vi "Configurator.vi"() -> ()   [LabVIEW 2017]
uses:
  Controls/Configurator Range Enum Type Def.ctl
  Controls/Configurator Rate Enum Type Def.ctl
  Controls/Configurator Resolution Enum Type Def.ctl
  Controls/Configurator State Type Def.ctl
panel:
  in  "Baud":bool=TRUE
  in  "First Erase?":bool=TRUE
  in  "VISA Port":refnum<visa-resource-name>="COM5"
  out "Error Out":errorcluster
  in  "Error In":errorcluster
  in  "Resolution":T1=enum."High Res (12 bit)"
  in  "ID":u8
  in  "Rate":T2
  in  "Range":T3=enum."±2g"
  # "Read and save measurement data before running this program!"
  # "6 Meg"
  # "3 Meg"
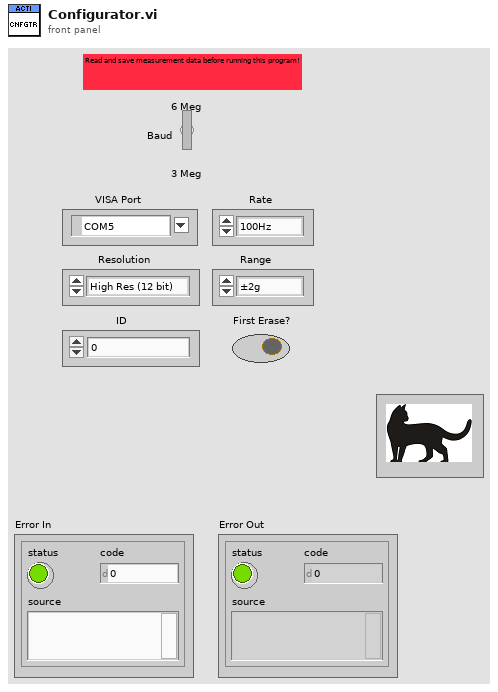
[diagram p1: front panel]
types:
  T1 = typedef "Configurator Resolution Enum Type Def.ctl" = enum16{"Low Res (10 bit)", "High Res (12 bit)"}
  T2 = typedef "Configurator Rate Enum Type Def.ctl" = enum16{"100Hz", "50Hz", "25Hz", "10Hz", "1Hz", "Idle"}
  T3 = typedef "Configurator Range Enum Type Def.ctl" = enum16{"±16g", "±8g", "±4g", "±2g"}
  T4 = typedef "Configurator State Type Def.ctl" = enum16{"Send Idle", "Send Time", "Construct Time String", "Close Serial", "Stop", "Error", "Dialog", "Start Measurement", "Chip Erase", "Send ID", "Send Range & Rate", "Construct Range Word", "Construct Rate Word", "Open Serial", "Latch Controls", "Init"}
  T5 = cluster{"Dialog?":bool, "Rate":T2, "Range":T3, "Resolution":T1, "ID":u8, "Range Word":u8, "Rate Word":u8, "Time Bytes":string, "VISA":refnum<visa-resource-name>, "First Erase?":bool, "Baud ":bool}
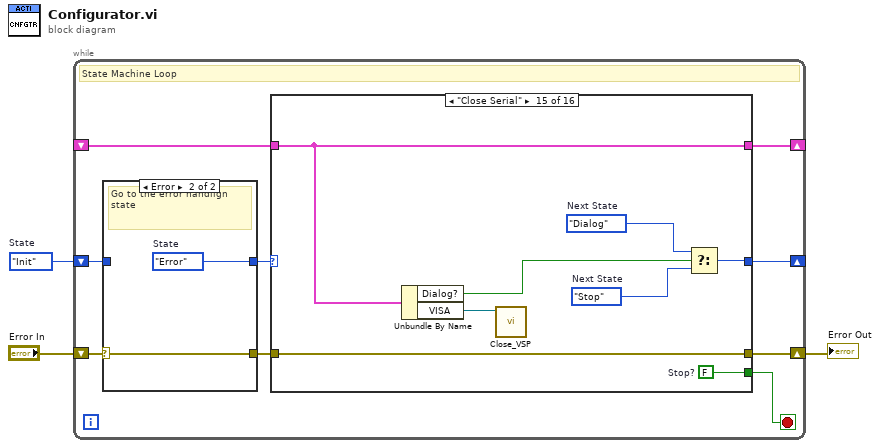
[diagram p0: block diagram]
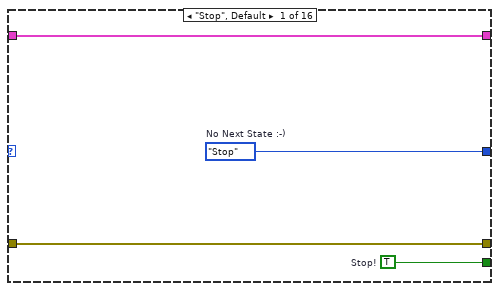
[diagram p2: hidden frame]
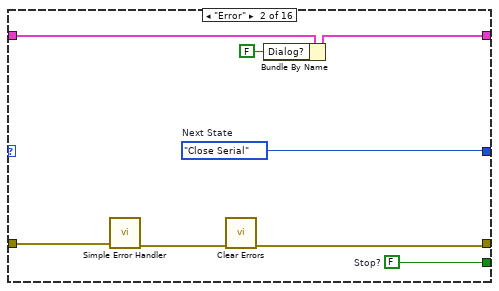
[diagram p3: hidden frame]
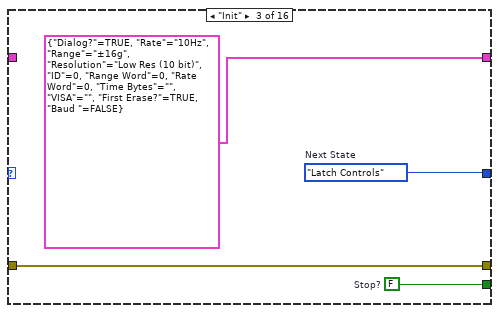
[diagram p4: hidden frame]
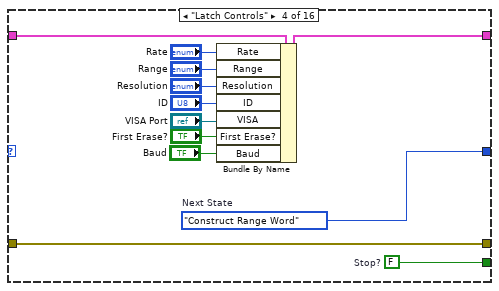
[diagram p5: hidden frame]
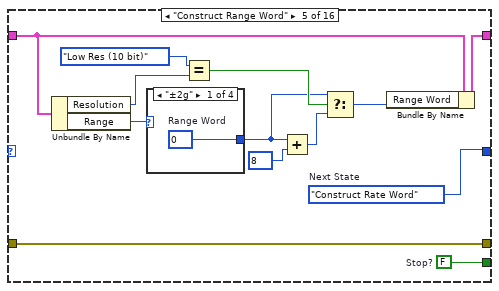
[diagram p6: hidden frame]
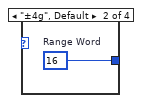
[diagram p7: hidden frame]
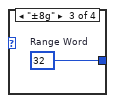
[diagram p8: hidden frame]
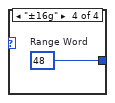
[diagram p9: hidden frame]
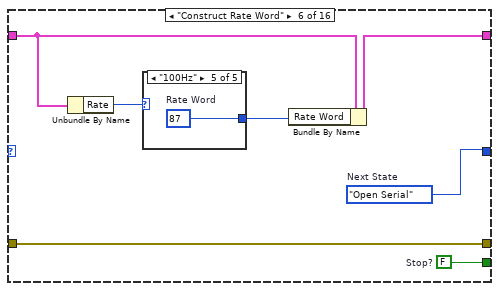
[diagram p10: hidden frame]
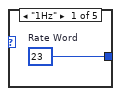
[diagram p11: hidden frame]
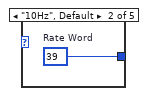
[diagram p12: hidden frame]
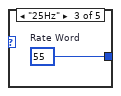
[diagram p13: hidden frame]
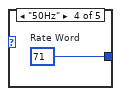
[diagram p14: hidden frame]
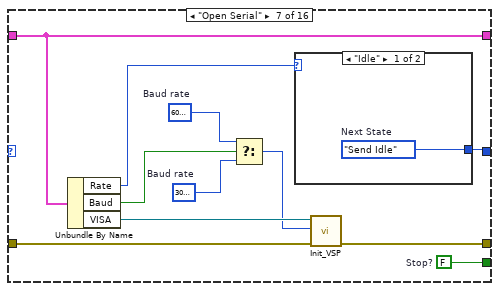
[diagram p15: hidden frame]
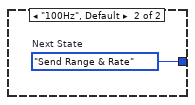
[diagram p16: hidden frame]
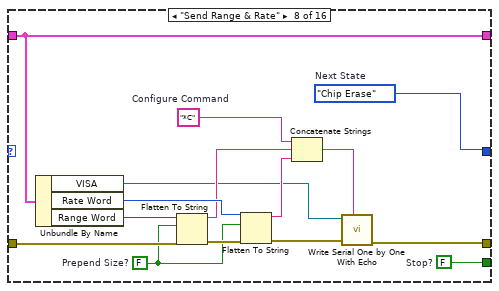
[diagram p17: hidden frame]
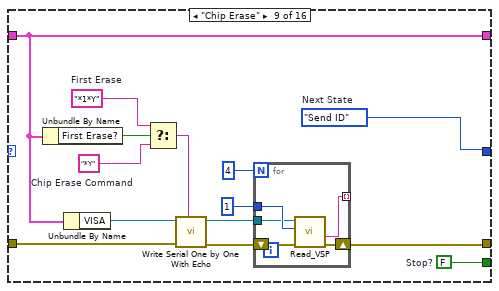
[diagram p18: hidden frame]
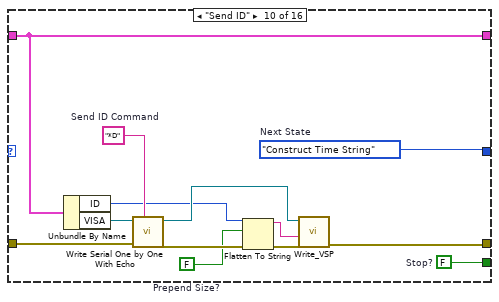
[diagram p19: hidden frame]
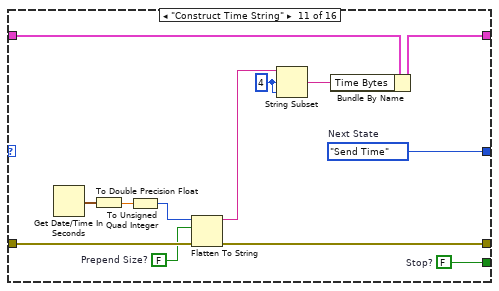
[diagram p20: hidden frame]
diagram:
  w2 = Configurator_State_Type_Def."Init"  # State
  n1 = while {
    shift-right: [w11] -> w1
    shift-left: "Error In" -> [w12]
    shift-right: [w8] -> _
    shift-left: w2 -> [w10]
    shift-right: [w6] -> _
    shift-left: _ -> [w5]
    stop <- w7 stop-if-true
    # "State Machine Loop"
    n2 = case shown="Error" w12 {
      selector: w12 -> [w192 w194]
      tunnel: [w192 w194] -> w4
      tunnel: w10 -> [w191 _]
      tunnel: [w191 w193] -> w9
      frame No Error {
        # "Go to next state"
      }
      frame Error {
        w193 = Configurator_State_Type_Def."Error"  # State
        # "Go to the error handlign state"
      }
    }
    n3 = case shown="\"Close Serial\"" w9 {
      tunnel: w4 -> [w16 w24 w25 w37 w52 w63 w78 w93 w109 w126 w137 w149 w156 w164 w175 w187]
      tunnel: [w16 w17 w25 w37 w52 w63 w77 w94 w107 w118 w136 w148 w155 w163 w175 w187] -> w11
      tunnel: [w15 w23 w28 w40 w50 w61 w79 w96 w110 w128 w141 w150 w157 w159 w177 w186] -> w8
      tunnel: [w14 w22 w27 w39 w53 w64 w80 w97 w111 w129 w142 w151 w158 FALSE ("Stop?") w182 w188] -> w7
      tunnel: [w13 w20 T5 {"Dialog?"=TRUE, "Rate"=enum."10Hz", "Range"=enum."±16g", "Resolution"=enum."Low Res (10 bit)", "ID"=0, "Range Word"=0, "Rate Word"=0, "Time Bytes"="", "VISA"="", "First Erase?"=TRUE, "Baud "=FALSE} w36 w42 w60 w76 w95 w99 w125 w133 w147 w154 w161 w181 w184] -> w6
      tunnel: w5 -> [w13 w21 _ w38 w51 w62 w76 w95 w99 w125 w140 w147 w154 w161 w181 w184]
      frame "Stop", Default {
        w14 = TRUE  # Stop!
        w15 = Configurator_State_Type_Def."Stop"  # No Next State :-)
      }
      frame "Error" {
        w22 = FALSE  # Stop?
        w23 = Configurator_State_Type_Def."Close Serial"  # Next State
        n4 = call <vilib>:"Simple Error Handler.vi"("error in (no error)"=w24) -> ("error out"=w18:errorcluster)  [unwired: 4 in, 4 out]
        n5 = call <vilib>:"Clear Errors.vi"("error in (no error)"=w18) -> ("error out"=w17:errorcluster)  [unwired: 5 in, 1 out]
        n6 = Bundle By Name(cluster=w21, "Dialog?"=FALSE) -> (w20:T5)
      }
      frame "Init" {
        w27 = FALSE  # Stop?
        w28 = Configurator_State_Type_Def."Latch Controls"  # Next State
      }
      frame "Latch Controls" {
        w39 = FALSE  # Stop?
        w40 = Configurator_State_Type_Def."Construct Range Word"  # Next State
        n7 = Bundle By Name(cluster=w38, "Rate"="Rate", "Range"="Range", "Resolution"="Resolution", "ID"="ID", "VISA"="VISA Port", "First Erase?"="First Erase?", "Baud"="Baud") -> (w36:T5)
      }
      frame "Construct Range Word" {
        w53 = FALSE  # Stop?
        w50 = Configurator_State_Type_Def."Construct Rate Word"  # Next State
        n8 = Unbundle By Name(w51) -> ("Resolution"=w46:T1, "Range"=w49:T3)
        n9 = case shown="\"±2g\"" w49 {
          tunnel: [w54 w55 w56 w57] -> w43
          frame "±2g" {
            w54 = u8 0  # Range Word
          }
          frame "±4g", Default {
            w55 = u8 16  # Range Word
          }
          frame "±8g" {
            w56 = u8 32  # Range Word
          }
          frame "±16g" {
            w57 = u8 48  # Range Word
          }
        }
        n10 = Equal?(x=Configurator_Resolution_Enum_Type_Def."Low Res (10 bit)" ("Resolution"), y=w46) -> (x = y?=w44:bool)
        n11 = Add(x=w43, y=u8 8) -> (x+y=w47:u8)
        n12 = Select(t=w43, s=w44, f=w47) -> (s? t:f=w41:u8)
        n13 = Bundle By Name(cluster=w51, "Range Word"=w41) -> (w42:T5)
      }
      frame "Construct Rate Word" {
        w64 = FALSE  # Stop?
        w61 = Configurator_State_Type_Def."Open Serial"  # Next State
        n14 = Unbundle By Name(w62) -> ("Rate"=w59:T2)
        n15 = case shown="\"100Hz\"" w59 {
          tunnel: [w65 w66 w67 w68 w69] -> w58
          frame "1Hz" {
            w65 = u8 23  # Rate Word
          }
          frame "10Hz", Default {
            w66 = u8 39  # Rate Word
          }
          frame "25Hz" {
            w67 = u8 55  # Rate Word
          }
          frame "50Hz" {
            w68 = u8 71  # Rate Word
          }
          frame "100Hz" {
            w69 = u8 87  # Rate Word
          }
        }
        n16 = Bundle By Name(cluster=w62, "Rate Word"=w58) -> (w60:T5)
      }
      frame "Open Serial" {
        w74 = u32 3000000  # Baud rate
        w73 = u32 6000000  # Baud rate
        w80 = FALSE  # Stop?
        n17 = Unbundle By Name(w76) -> ("Rate"=w70:T2, "Baud"=w71:bool, "VISA"=w75:refnum<visa-resource-name>)
        n18 = Select(t=w73, s=w71, f=w74) -> (s? t:f=w72:u32)
        n19 = case shown="\"Idle\"" w70 {
          tunnel: [w81 w82] -> w79
          frame "Idle" {
            w81 = Configurator_State_Type_Def."Send Idle"  # Next State
          }
          frame "100Hz", Default {
            w82 = Configurator_State_Type_Def."Send Range & Rate"  # Next State
          }
        }
        n20 = call "Init_VSP.vi"("error in"=w78, "Baud rate"=w72, "VISA resource name"=w75) -> ("error out"=w77:errorcluster)  [unwired: 7 in, 1 out]
      }
      frame "Send Range & Rate" {
        w89 = FALSE  # Prepend Size?
        w87 = "*C"  # Configure Command
        w97 = FALSE  # Stop?
        w96 = Configurator_State_Type_Def."Chip Erase"  # Next State
        n21 = Unbundle By Name(w95) -> ("VISA"=w84:refnum<visa-resource-name>, "Rate Word"=w88:u8, "Range Word"=w90:u8)
        n22 = Flatten To String(anything=w90, prepend array or string size? (T)=w89, error in (no error)=w93) -> (data string=w86:string, error out=w92:errorcluster)  [unwired: 1 in, 1 out]
        n23 = Flatten To String(anything=w88, prepend array or string size? (T)=w89, error in (no error)=w92) -> (data string=w85:string, error out=w91:errorcluster)  [unwired: 1 in, 1 out]
        n24 = Concatenate Strings(w87, w86, w85) -> (w83:string)
        n25 = call "Write Serial One by One With Echo.vi"("String"=w83, "Error In"=w91, "VISA In"=w84) -> ("Error Out"=w94:errorcluster)  [unwired: 7 in, 1 out]
      }
      frame "Chip Erase" {
        w103 = "*1*Y"  # First Erase
        w102 = "*Y"  # Chip Erase Command
        w111 = FALSE  # Stop?
        w110 = Configurator_State_Type_Def."Send ID"  # Next State
        n26 = Unbundle By Name(w99) -> ("First Erase?"=w98:bool)
        n27 = Unbundle By Name(w99) -> ("VISA"=w101:refnum<visa-resource-name>)
        n28 = Select(t=w103, s=w98, f=w102) -> (s? t:f=w100:string)
        n29 = call "Write Serial One by One With Echo.vi"("String"=w100, "Error In"=w109, "VISA In"=w101) -> ("Error Out"=w108:errorcluster, "VISA Out"=w105:refnum<visa-resource-name>)  [unwired: 7 in]
        n30 = for {
          N: 4 -> [_]
          shift-right: [w115] -> w107
          shift-left: w108 -> [w116]
          tunnel: u32 1 ("Requested byte cout") -> [w114]
          tunnel: w105 -> [w113]
          tunnel: [w112] -> _ mode=indexing
          n31 = call "Read_VSP.vi"("error in"=w116, "Requested byte cout"=w114, "VISA resource name"=w113) -> ("error out"=w115:errorcluster, "String"=w112:string)  [unwired: 1 in, 2 out]
        }
      }
      frame "Send ID" {
        w122 = FALSE  # Prepend Size?
        w127 = "*D"  # Send ID Command
        w129 = FALSE  # Stop?
        w128 = Configurator_State_Type_Def."Construct Time String"  # Next State
        n32 = Unbundle By Name(w125) -> ("ID"=w117:u8, "VISA"=w124:refnum<visa-resource-name>)
        n33 = call "Write Serial One by One With Echo.vi"("String"=w127, "Error In"=w126, "VISA In"=w124) -> ("Error Out"=w123:errorcluster, "VISA Out"=w120:refnum<visa-resource-name>)  [unwired: 7 in]
        n34 = Flatten To String(anything=w117, prepend array or string size? (T)=w122, error in (no error)=w123) -> (data string=w119:string, error out=w121:errorcluster)  [unwired: 1 in, 1 out]
        n35 = call "Write_VSP.vi"("error in"=w121, "String"=w119, "VISA resource name"=w120) -> ("error out"=w118:errorcluster)  [unwired: 2 in, 2 out]
      }
      frame "Construct Time String" {
        w130 = 4 ("offset (0)")
        w134 = FALSE  # Prepend Size?
        w142 = FALSE  # Stop?
        w141 = Configurator_State_Type_Def."Send Time"  # Next State
        n36 = Get Date/Time In Seconds() -> (seconds since 1Jan1904=w139:timestamp)
        n37 = To Double Precision Float(number=w139) -> (double precision float=w138:dbl)
        n38 = To Unsigned Quad Integer(1:w138) -> (0:w135:u64)
        n39 = Flatten To String(anything=w135, prepend array or string size? (T)=w134, error in (no error)=w137) -> (data string=w131:string, error out=w136:errorcluster)  [unwired: 1 in, 1 out]
        n40 = String Subset(string=w131, offset (0)=w130, length (rest)=w130) -> (substring=w132:string)
        n41 = Bundle By Name(cluster=w140, "Time Bytes"=w132) -> (w133:T5)
      }
      frame "Send Time" {
        w146 = "*T"  # Set Time Command
        w151 = FALSE  # Stop?
        w150 = Configurator_State_Type_Def."Start Measurement"  # Next State
        n42 = Unbundle By Name(w147) -> ("Time Bytes"=w145:string, "VISA"=w144:refnum<visa-resource-name>)
        n43 = Concatenate Strings(w146, w145) -> (w143:string)
        n44 = call "Write Serial One by One With Echo.vi"("String"=w143, "Error In"=w149, "VISA In"=w144) -> ("Error Out"=w148:errorcluster)  [unwired: 7 in, 1 out]
      }
      frame "Start Measurement" {
        w152 = "*S"  # Start Command
        w158 = FALSE  # Stop?
        w157 = Configurator_State_Type_Def."Close Serial"  # Next State
        n45 = Unbundle By Name(w154) -> ("VISA"=w153:refnum<visa-resource-name>)
        n46 = call "Write Serial One by One With Echo.vi"("String"=w152, "Error In"=w156, "VISA In"=w153) -> ("Error Out"=w155:errorcluster)  [unwired: 7 in, 1 out]
      }
      frame "Send Idle" {
        w159 = Configurator_State_Type_Def."Close Serial"  # Next State
        w167 = u32 1  # Requested byte cout
        n47 = Unbundle By Name(w161) -> ("VISA"=w160:refnum<visa-resource-name>)
        n48 = call "Write_VSP.vi"("error in"=w164, "String"="*", "VISA resource name"=w160) -> ("error out"=w173:errorcluster, "duplicate VISA resource name"=w172:refnum<visa-resource-name>)  [unwired: 2 in, 1 out]
        n49 = call "Read_VSP.vi"("error in"=w173, "Requested byte cout"=w167, "VISA resource name"=w172) -> ("error out"=w169:errorcluster, "duplicate VISA resource name"=w168:refnum<visa-resource-name>)  [unwired: 1 in, 2 out]
        n50 = Flatten To String(anything=u8 27) -> (data string=w165:string)  [unwired: 3 in, 2 out]
        n51 = call "Write_VSP.vi"("error in"=w169, "String"=w165, "VISA resource name"=w168) -> ("error out"=w170:errorcluster, "duplicate VISA resource name"=w171:refnum<visa-resource-name>)  [unwired: 2 in, 1 out]
        n52 = call "Read_VSP.vi"("error in"=w170, "Requested byte cout"=w167, "VISA resource name"=w171) -> ("error out"=w163:errorcluster)  [unwired: 1 in, 3 out]
      }
      frame "Close Serial" {
        w179 = Configurator_State_Type_Def."Stop"  # Next State
        w182 = FALSE  # Stop?
        w178 = Configurator_State_Type_Def."Dialog"  # Next State
        n53 = Unbundle By Name(w181) -> ("Dialog?"=w176:bool, "VISA"=w180:refnum<visa-resource-name>)
        n54 = call "Close_VSP.vi"("VISA resource name"=w180) -> ()  [unwired: 6 in, 1 out]
        n55 = Select(t=w178, s=w176, f=w179) -> (s? t:f=w177:T4)
      }
      frame "Dialog" {
        w186 = Configurator_State_Type_Def."Stop"  # Next State
        w188 = FALSE  # Stop?
        n56 = Unbundle By Name(w184) -> ("Rate"=w185:T2)
        n57 = case shown="\"Idle\"" w185 {
          tunnel: ["Idle command sent.\nRemove device now." ("message") "Start command sent.\nRemove device now." ("message")] -> w183
          frame "Idle" {
          }
          frame "100Hz", Default {
          }
        }
        n58 = One Button Dialog(message=w183) -> ()  [unwired: 1 in, 1 out]
      }
    }
  }
  "Error Out" <- w1
